vi "Microchip 93C86 Read.vi"() -> ()   [LabVIEW 2015]
doc: "This example shows a more generalized way to use the SPI advanced API to read data. It allows the user to change the following parameters: the endianness of the address bytes, and the number of bytes in an address.\n\nThe parameters will have the following effects:\n\nData Address Width: This will allow the user to specify the EEPROM Data Address as either 1 or 2 bytes.\nData Address Endianness: This control will change the ordering of the bytes in the EEPROM Data Address, note that this only has an effect if there are 2 bytes in the address.\n\nFor connection information see the NI-845x Hardware and Software manual and the manual for your specific SPI device."
uses:
  <vilib>/ni845x/ni845x.llb/ni845xControl.ctl
  <vilib>/ni845x/ni845x.llb/NI-845x SPI Close Script Reference.vi
  <resource>/objmgr/NI845x.rc
panel:
  in  "Target Page Size (bytes)":u32=2
  in  "I/O Voltage Level":i32(ring)=33 items=["3.3V"=33, "2.5V"=25, "1.8V"=18, "1.5V"=15, "1.2V"=12]
  in  "Data Address Width":enum16{"1 Byte", "2 Byte"}(ring)=enum."2 Byte"
  in  "Data Address Endianness":bool=TRUE
  in  "EEPROM Data Address":u8 format="%.0x"
  in  "Number of Bytes to Read":u32=2
  in  "Clock Rate (kHz)":u16=2000
  in  "Chip Select":u32
  out "Read Data":u16[](array[numeric]) format="%x"
  in  "Device":T1="NI-8451"
  # "Device Configuration"
  # "SPI Data"
  # "SPI Slave Configuration"
  # "Note 1: Microchip 93C76/86\nEEPROM devices DC signal levels\nare 2.0V (min) to Vcc (5.0V) +1V\nmax.\n\nNote 2: NI-8451 max signal\nlevel is 3.5V so recommended\nI/O voltage of 3.3V is OK."
  # "Big Endian"
  # "Little Endian"
  # "2048 x 8- or 1024 x 16-bit organization (93C86)"
  # "Clock frequency FCLK — 2 MHz"
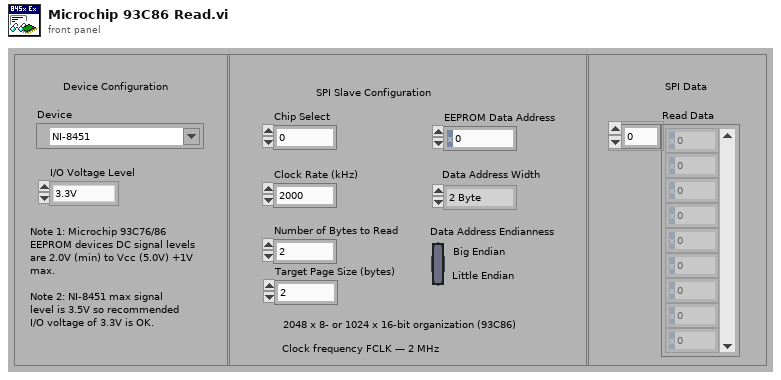
[diagram p1: front panel]
types:
  T1 = typedef "ni845xControl.ctl" = refnum<k21>
  T2 = typedef "ni845xSpiScriptControl.ctl" = refnum<k20>
  T3 = cluster{"EEPROM Address":u16, "Length":u32, "Data Index":u32}[]
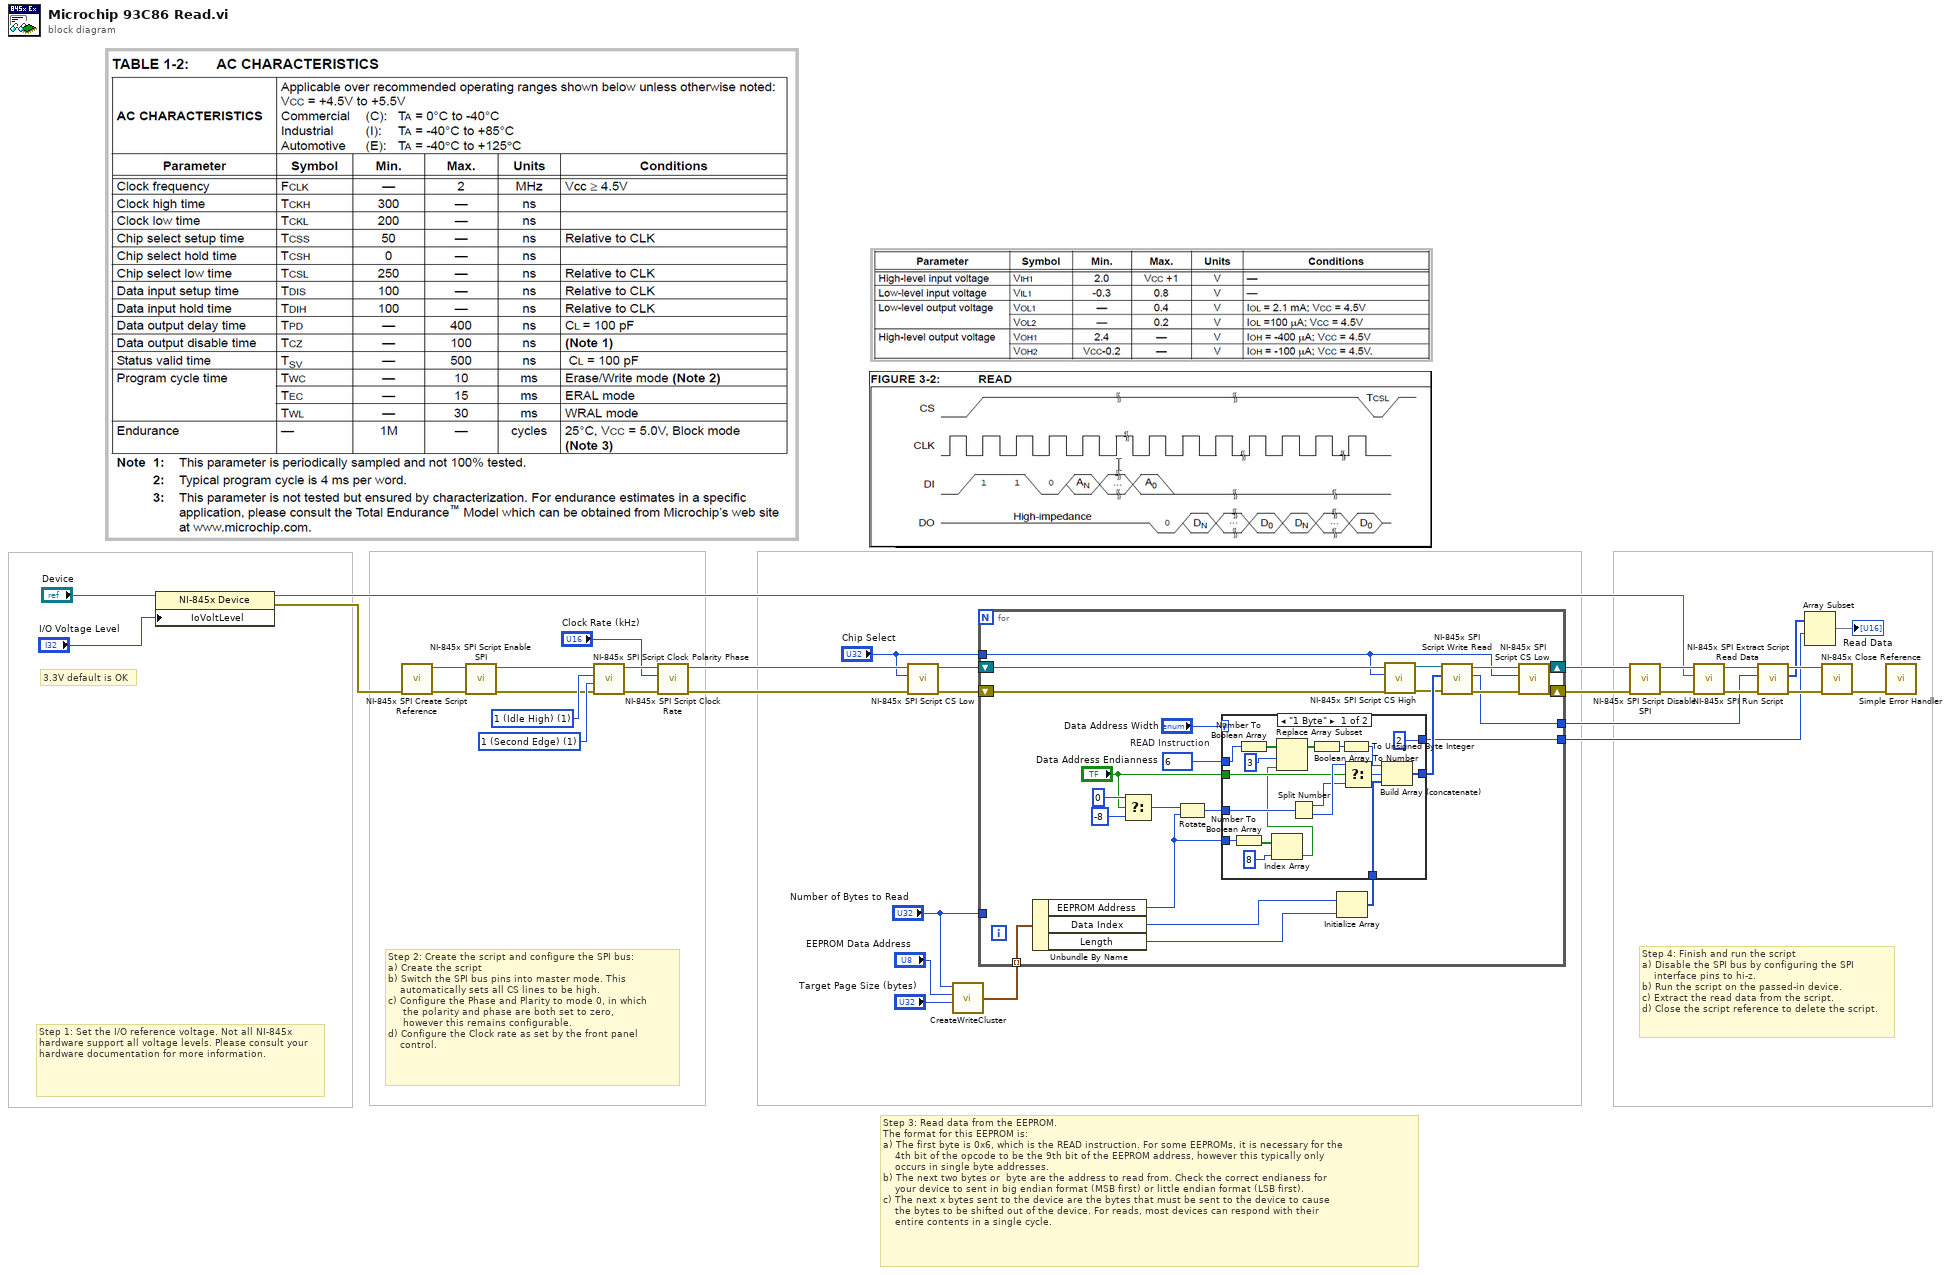
[diagram p0: block diagram]
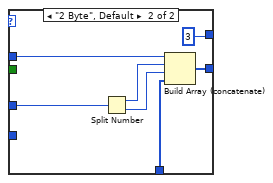
[diagram p2: hidden frame]
diagram:
  w22 = 1 items=["0 (First Edge)", "1 (Second Edge)"] ("clock phase (0)")
  w23 = 1 items=["0 (Idle Low)", "1 (Idle High)"] ("clock polarity (0)")
  # "3.3V default is OK"
  # "Step 1: Set the I/O reference voltage. Not all NI-845x hardware support all voltage levels. Please consult your hardware documentation for more information."
  # "Step 4: Finish and run the script\na) Disable the SPI bus by configuring the SPI \n    interface pins to hi-z.\nb) Run the script on the passed-in device. \nc) Extract the read data from the script.\nd) Close the script reference to delete the script."
  # "Step 3: Read data from the EEPROM. \nThe format for this EEPROM is:\na) The first byte is 0x6, which is the READ instruction. For some EEPROMs, it is necessary for the   \n    4th bit of the opcode to be the 9th bit of the EEPROM address, however this typically only   \n    occurs in single byte addresses.\nb) The next two bytes or  byte are the address to read from. Check the correct endianess for\n    your device to sent in big endian format (MSB first) or little endian format (LSB first).\nc) The next x bytes sent to the device are the bytes that must be sent to the device to cause \n    the bytes to be shifted out of the device. For reads, most devices can respond with their \n    entire contents in a single cycle."
  # "Step 2: Create the script and configure the SPI bus:\na) Create the script\nb) Switch the SPI bus pins into master mode. This\n    automatically sets all CS lines to be high.\nc) Configure the Phase and Plarity to mode 0, in which \n     the polarity and phase are both set to zero,\n     however this remains configurable. \nd) Configure the Clock rate as set by the front panel \n    control."
  n1 = property on="Property Node" class="NI-845x Device"(reference="Device", "IoVoltLevel"="I/O Voltage Level") -> (reference out=w10:T1, error out=w9:errorcluster)  [unwired: 1 in]
  n2 = call <vilib>:"NI-845x SPI Create Script Reference.vi"("error in (no error)"=w9) -> ("error out"=w20:errorcluster, "spi script reference"=w21:T2)  [unwired: 9 out]
  n3 = call <vilib>:"NI-845x SPI Script Enable SPI.vi"("error in (no error)"=w20, "spi script reference in"=w21) -> ("error out"=w18:errorcluster, "spi script reference out"=w19:T2)  [unwired: 8 out]
  n4 = call <vilib>:"NI-845x SPI Script Clock Polarity Phase.vi"("error in (no error)"=w18, "clock phase (0)"=w22, "clock polarity (0)"=w23, "spi script reference in"=w19) -> ("error out"=w33:errorcluster, "spi script reference out"=w32:T2)  [unwired: 2 in, 4 out]
  n5 = call <vilib>:"NI-845x SPI Script Clock Rate.vi"("error in (no error)"=w33, "clock rate in kHz (1000)"="Clock Rate (kHz)", "spi script reference in"=w32) -> ("error out"=w28:errorcluster, "spi script reference out"=w27:T2)  [unwired: 1 in, 6 out]
  n6 = call <vilib>:"NI-845x SPI Script CS Low.vi"("error in (no error)"=w28, "chip select (0)"="Chip Select", "spi script reference in"=w27) -> ("error out"=w7:errorcluster, "spi script reference out"=w6:T2)  [unwired: 1 in, 6 out]
  n7 = call "CreateWriteCluster.vi"("Page Size in Bytes"="Target Page Size (bytes)", "EEPROM Starting Address"="EEPROM Data Address", "Number of Bytes to Write"="Number of Bytes to Read") -> ("Array of Write Cluster Information"=w1:T3)  [unwired: 1 in]
  n8 = for {
    tunnel: [w55] -> w24
    tunnel: [w45] -> w12
    tunnel: "Chip Select" -> [w40]
    tunnel: "Number of Bytes to Read" -> [_]
    shift-right: [w59] -> w34
    shift-left: w7 -> [w44]
    shift-right: [w56] -> w31
    shift-left: w6 -> [w43]
    tunnel: w1 -> [w39] mode=indexing
    w51 = u8 6  # READ Instruction
    n9 = Unbundle By Name(w39) -> ("EEPROM Address"=w38:u16, "Data Index"=w37:u32, "Length"=w36:u32)
    n10 = Select(t=i16 0, s="Data Address Endianness", f=i16 -8) -> (s? t:f=w52:i16)
    n11 = Rotate(1:w38, 2:w52) -> (0:w49:u16)
    n12 = Initialize Array(w37, w36) -> (w46:u32[])
    n13 = case shown="\"1 Byte\"" "Data Address Width" {
      tunnel: w49 -> [w76 w82]
      tunnel: [w77 w79] -> w47
      tunnel: w51 -> [w71 w81]
      tunnel: "Data Address Endianness" -> [w72 _]
      tunnel: w46 -> [w65 w80]
      tunnel: [2 ("index") 3 ("index")] -> w45
      tunnel: w38 -> [w61 _]
      frame "1 Byte" {
        n14 = Number To Boolean Array(number=w61) -> (Boolean array=w63:bool[])
        n15 = Number To Boolean Array(number=w71) -> (Boolean array=w70:bool[])
        n16 = Index Array(array=w63, index=8) -> (element=w62:bool)
        n17 = Replace Array Subset(array=w70, new element=w62, index=3) -> (w68:bool[])
        n18 = Split Number(x=w76) -> (hi(x)=w74:u8, lo(x)=w75:u8)
        n19 = Boolean Array To Number(Boolean array=w68) -> (number=w67:u32)
        n20 = To Unsigned Byte Integer(number=w67) -> (unsigned 8bit integer=w66:u8)
        n21 = Select(t=w75, s=w72, f=w74) -> (s? t:f=w73:u8)
        n22 = Build Array (concatenate)(w66, w73, w65) -> (w77:u32[])
      }
      frame "2 Byte", Default {
        n23 = Split Number(x=w82) -> (hi(x)=w84:u8, lo(x)=w83:u8)
        n24 = Build Array (concatenate)(w81, w84, w83, w80) -> (w79:u32[])
      }
    }
    n25 = call <vilib>:"NI-845x SPI Script CS High.vi"("error in (no error)"=w44, "chip select (0)"=w40, "spi script reference in"=w43) -> ("error out"=w42:errorcluster, "spi script reference out"=w41:T2)  [unwired: 7 in]
    n26 = call <vilib>:"NI-845x SPI Script Write Read.vi"("error in (no error)"=w42, "write data"=w47, "spi script reference in"=w41) -> ("error out"=w58:errorcluster, "script read index"=w55:u32, "spi script reference out"=w57:T2)  [unwired: 1 in, 5 out]
    n27 = call <vilib>:"NI-845x SPI Script CS Low.vi"("error in (no error)"=w58, "chip select (0)"=w40, "spi script reference in"=w57) -> ("error out"=w59:errorcluster, "spi script reference out"=w56:T2)  [unwired: 7 in]
  }
  n28 = call <vilib>:"NI-845x SPI Script Disable SPI.vi"("error in (no error)"=w34, "spi script reference in"=w31) -> ("error out"=w35:errorcluster, "spi script reference out"=w30:T2)  [unwired: 8 out]
  n29 = call <vilib>:"NI-845x SPI Run Script.vi"("error in (no error)"=w35, "device reference in"=w10, "spi script reference in"=w30) -> ("error out"=w26:errorcluster, "spi script reference out"=w25:T2)  [unwired: 1 in, 6 out]
  n30 = call <vilib>:"NI-845x SPI Extract Script Read Data.vi"("error in (no error)"=w26, "script read index"=w24, "spi script reference in"=w25) -> ("error out"=w16:errorcluster, "read data"=w13:u8[], "spi script reference out"=w17:T2)  [unwired: 6 out]
  n31 = Array Subset(array=w13, index=w12) -> (→"Read Data":u8[])  [unwired: 1 in]
  n32 = call-poly <vilib>:"NI-845x Close Reference.vi"("error in (no error)"=w16, "spi script reference"=w17) -> ("error out"=w15:errorcluster)  [unwired: 9 out]
  n33 = call <vilib>:"Simple Error Handler.vi"("error in (no error)"=w15) -> ()  [unwired: 1 in, 8 out]
